vi "message.vi"(2 "error in (no error)":errorcluster, 3 "msgop":i32(ring) items=["0"=0, "1"=1, "6"=6, "7"=7, "8"=8, "9"=9], 4 "retcode":u16(ring) items=["0"=0, "1"=1, "100"=100, "101"=101, "102"=102, "200"=200, "201"=202, "300"=300, "301"=301, "302"=302, "303"=303, "304"=304, "305"=305, "306"=306, "307"=307, "308"=308, "309"=309, "400"=400, "500"=500, "501"=501, "502"=502, "999"=999], 5 "msgtype":i32(ring) items=["2"=2, "3"=3, "4"=4], 6 "lockout_key":string, 7 "input json string":string) -> (0 "error out":errorcluster, 1 "body":string)   [LabVIEW 2016]
doc: "Format the message to follow dripline standard"
panel:
  in  "return_msg":string
  out "sender_info":T1
  out "timestamp":string
  in  "package":string="dripline"
  in  "commit":string="xxxxx"
  in  "version":string="v0.0.0"
  in  "service_name":string="dripline"
  out "exe":string
  out "username":string
  out "hostname":string
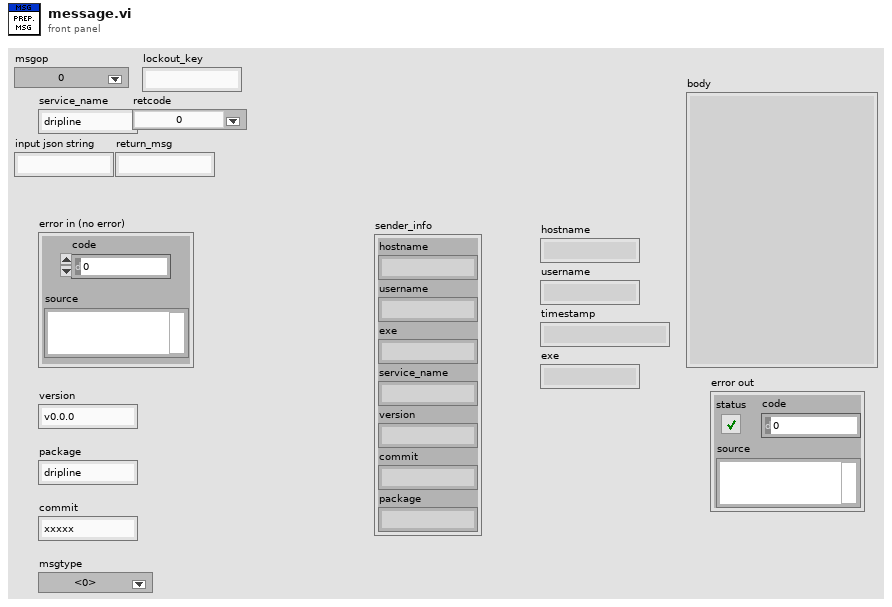
[diagram p1: front panel]
types:
  T1 = cluster{"hostname":string, "username":string, "exe":string, "service_name":string, "version":string, "commit":string, "package":string}
  T2 = cluster{"sender_info":string, "timestamp":string, "input":string}
  T3 = cluster{"timestamp":string, "retcode":u16, "return_msg":string, "sender_info":cluster{"hostname":string, "username":string, "exe":string, "service_name":string, "version":string, "commit":string, "package":string}, "msgtype":i32}
  T4 = cluster{"lockout_key":string, "timestamp":string, "msgop":i32, "sender_info":cluster{"hostname":string, "username":string, "exe":string, "service_name":string, "version":string, "commit":string, "package":string}, "msgtype":i32}
  T5 = cluster{"timestamp":string, "sender_info":cluster{"hostname":string, "username":string, "exe":string, "service_name":string, "version":string, "commit":string, "package":string}, "msgtype":i32}
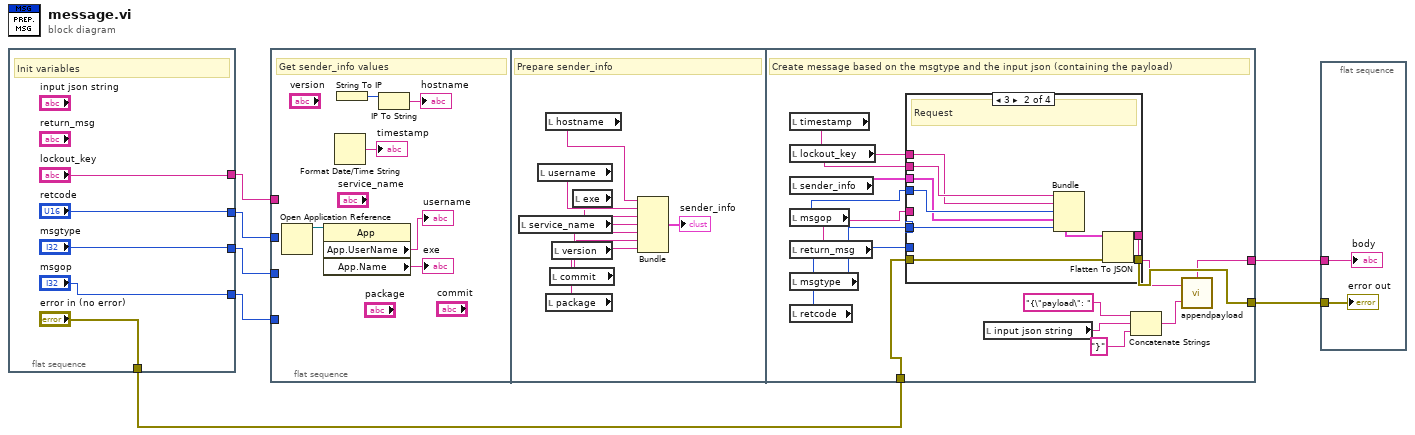
[diagram p0: block diagram]
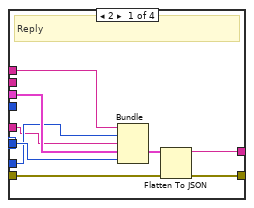
[diagram p2: hidden frame]
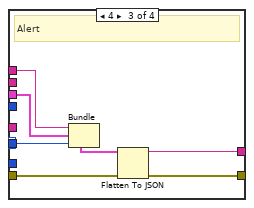
[diagram p3: hidden frame]
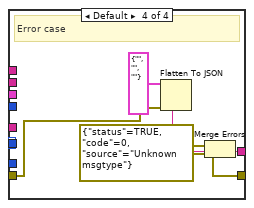
[diagram p4: hidden frame]
diagram:
  n1 = flat-sequence {
    tunnel: ["msgtype"] -> w6
    tunnel: ["error in (no error)"] -> w4
    tunnel: ["msgop"] -> w3
    tunnel: ["lockout_key"] -> w2
    tunnel: ["retcode"] -> w1
    frame #0 {
      # "Init variables"
    }
  }
  n2 = flat-sequence {
    tunnel: w6 -> [_]
    tunnel: w3 -> [_]
    tunnel: w2 -> [_]
    tunnel: w1 -> [_]
    tunnel: [w40] -> w7
    tunnel: [w32] -> w5
    tunnel: w4 -> [w38]
    frame #0 {
      # "Get sender_info values"
      n3 = Open Application Reference() -> (3:w15:refnum<vi>)  [unwired: 4 in, 1 out]
      n4 = property class="App"(reference=w15) -> ("App.UserName"=→"username":string, "App.Name"=→"exe":string)  [unwired: 1 in, 2 out]
      n5 = Format Date/Time String() -> (date/time string=→"timestamp":string)  [unwired: 3 in]
      n6 = String To IP() -> (0:w16:u32)  [unwired: 1 in]
      n7 = IP To String(2:w16) -> (0:→"hostname":string)  [unwired: 1 in]
    }
    frame #1 {
      # "Prepare sender_info"
      n8 = local read "service_name"() -> (w23:string)
      n9 = local read "username"() -> (w26:string)
      n10 = local read "hostname"() -> (w25:string)
      n11 = local read "package"() -> (w20:string)
      n12 = local read "commit"() -> (w21:string)
      n13 = local read "version"() -> (w22:string)
      n14 = local read "exe"() -> (w24:string)
      n15 = Bundle("hostname"=w25, "username"=w26, "exe"=w24, "service_name"=w23, "version"=w22, "commit"=w21, "package"=w20) -> (→"sender_info":T1)  [unwired: 1 in]
    }
    frame #2 {
      # "Create message based on the msgtype and the input json (containing the payload)"
      n16 = local read "timestamp"() -> (w41:string)
      n17 = local read "lockout_key"() -> (w36:string)
      n18 = local read "sender_info"() -> (w39:T1)
      n19 = local read "msgop"() -> (w37:i32)
      n20 = local read "return_msg"() -> (w31:string)
      n21 = local read "msgtype"() -> (w34:i32)
      n22 = local read "retcode"() -> (w35:u16)
      n23 = case shown="3" w34 {
        tunnel: w41 -> [w47 w55 w63 _]
        tunnel: w38 -> [w49 w59 w66 w70]
        tunnel: [w48 w58 w64 w68] -> w40
        tunnel: [w50 w57 w65 w71] -> w33
        tunnel: w39 -> [w46 w53 w62 _]
        tunnel: w37 -> [_ w54 _ _]
        tunnel: w36 -> [_ w56 _ _]
        tunnel: w35 -> [w44 _ _ _]
        tunnel: w34 -> [w45 w52 w61 _]
        tunnel: w31 -> [w43 _ _ _]
        frame 2 {
          # "Reply"
          n24 = Bundle("timestamp"=w47, "retcode"=w44, "return_msg"=w43, "sender_info"=w46, "msgtype"=w45) -> (w42:T3)  [unwired: 1 in]
          n25 = Flatten To JSON(anything=w42, error in (no error)=w49) -> (JSON string=w50:string, 11:w48:errorcluster)  [unwired: 1 in]
        }
        frame 3 {
          # "Request"
          n26 = Bundle("lockout_key"=w56, "timestamp"=w55, "msgop"=w54, "sender_info"=w53, "msgtype"=w52) -> (w51:T4)  [unwired: 1 in]
          n27 = Flatten To JSON(anything=w51, error in (no error)=w59) -> (JSON string=w57:string, 11:w58:errorcluster)  [unwired: 1 in]
        }
        frame 4 {
          # "Alert"
          n28 = Bundle("timestamp"=w63, "sender_info"=w62, "msgtype"=w61) -> (w60:T5)  [unwired: 1 in]
          n29 = Flatten To JSON(anything=w60, error in (no error)=w66) -> (JSON string=w65:string, 11:w64:errorcluster)  [unwired: 1 in]
        }
        frame Default {
          # "Error case"
          n30 = Flatten To JSON(anything=T2 {"sender_info"="", "timestamp"="", "input"=""}, error in (no error)=w70) -> (JSON string=w71:string, 11:w69:errorcluster)  [unwired: 1 in]
          n31 = Merge Errors(w69, errorcluster {"status"=TRUE, "code"=0, "source"="Unknown msgtype"} ("error constant")) -> (w68:errorcluster)
        }
      }
      n32 = local read "input json string"() -> (w27:string)
      n33 = Concatenate Strings("{\"payload\": " ("string"), w27, "}" ("string")) -> (w28:string)
      n34 = call "appendpayload.vi"("jsontoappend"=w28, "basejson"=w33) -> ("concatenated json string"=w32:string)
    }
  }
  n35 = flat-sequence {
    tunnel: w7 -> [w74]
    tunnel: w5 -> [w73]
    frame #0 {
      "error out" <- w74
      "body" <- w73
    }
  }
